vi "IntegStart.vi"(0 "Time step":dbl format="%#_13g", 1 "Generator frequency":dbl, 2 "Number of ignored periods":i32, 3 "Field":dbl[](array[numeric]), 4 "BH averages":i32) -> (5 "Min Index":i32[](array[numeric]), 6 "Max Index":i32[](array[numeric]))   [LabVIEW 2015]
uses:
  <vilib>/express/express arith-compare/Formula/XNode/ExpressFormulaBlockNode.xnode
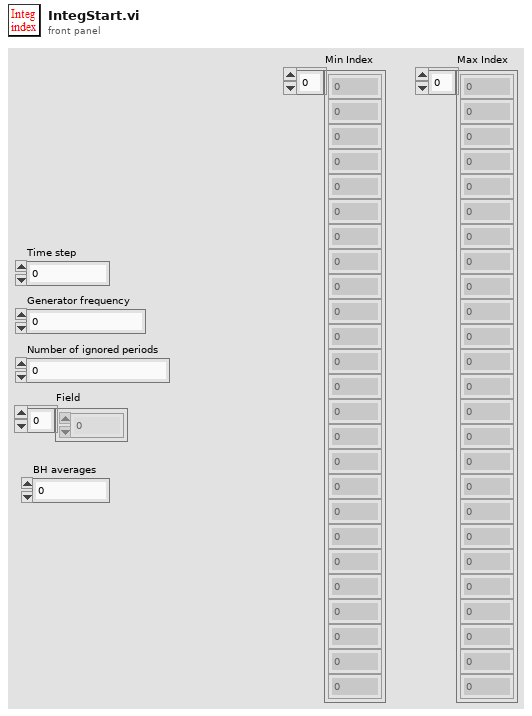
[diagram p1: front panel]
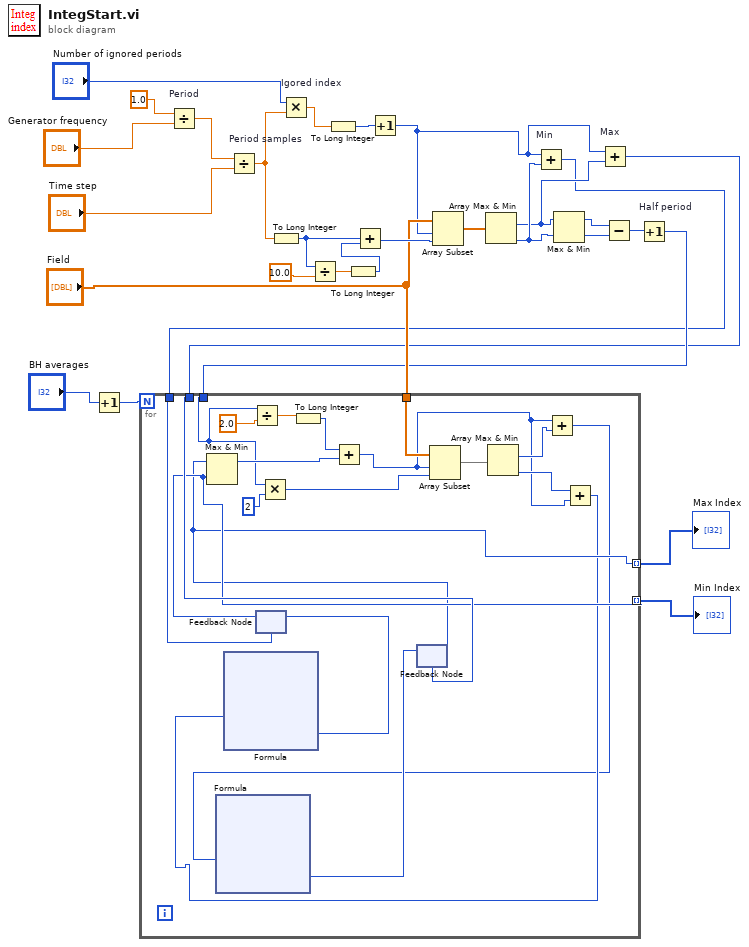
[diagram p0: block diagram]
diagram:
  n1 = Increment(x="BH averages") -> (x+1=w5:i32)
  n2 = Divide "Period"(x=1.0, y="Generator frequency") -> (x/y=w18:dbl)
  n3 = Divide "Period samples"(x=w18, y="Time step") -> (x/y=w19:dbl)
  n4 = To Long Integer(number=w19) -> (32bit integer=w16:i32)
  n5 = Multiply "Igored index"(x="Number of ignored periods", y=w19) -> (x*y=w23:dbl)
  n6 = Divide(x=w16, y=10.0) -> (x/y=w15:dbl)
  n7 = To Long Integer(number=w23) -> (32bit integer=w20:i32)
  n8 = To Long Integer(number=w15) -> (32bit integer=w14:i32)
  n9 = Add(x=w16, y=w14) -> (x+y=w13:i32)
  n10 = Increment(x=w20) -> (x+1=w9:i32)
  n11 = Array Subset(array="Field", index=w9, length=w13) -> (w24:dbl[])
  n12 = Array Max & Min(array=w24) -> (max index (indices)=w8:i32, min index (indices)=w10:i32)  [unwired: 2 out]
  n13 = Add "Min"(x=w9, y=w10) -> (x+y=w2:i32)
  n14 = Max & Min(x=w8, y=w10) -> (max(x,y)=w22:i32, min(x,y)=w21:i32)
  n15 = Add "Max"(x=w9, y=w8) -> (x+y=w1:i32)
  n16 = Subtract(x=w22, y=w21) -> (x-y=w12:i32)
  n17 = Increment "Half period"(x=w12) -> (x+1=w3:i32)
  n18 = for {
    N: w5 -> [_]
    tunnel: "Field" -> [w48]
    tunnel: [w32] -> w6 mode=indexing
    tunnel: [w31] -> w7 mode=indexing
    tunnel: w3 -> [w40]
    tunnel: w1 -> [w33]
    tunnel: w2 -> [w35]
    n19 = Divide(x=w40, y=2.0) -> (x/y=w45:dbl)
    n20 = feedback #1(w35) -> (w32:i32)
    n21 = Multiply(x=w40, y=2) -> (x*y=w42:i32)
    n22 = To Long Integer(number=w45) -> (32bit integer=w44:i32)
    n23 = feedback #2(w33) -> (w31:i32)
    n24 = Max & Min(x=w31, y=w32) -> (max(x,y)=w41:i32)  [unwired: 1 out]
    n25 = Add(x=w44, y=w41) -> (x+y=w37:i32)
    n26 = Array Subset(array=w48, index=w37, length=w42) -> (w47:dbl[])
    n27 = Array Max & Min(array=w47) -> (max index (indices)=w39:i32, min index (indices)=w38:i32)  [unwired: 2 out]
    n28 = Add(x=w37, y=w39) -> (x+y=w29:i32)
    n29 = xnode "Formula"("X1"=w29) -> ("Result"=w34:i32)  [unwired: 1 in, 1 out]
    n30 = feedback-in #2(w34) -> ()
    n31 = Add(x=w38, y=w37) -> (x+y=w30:i32)
    n32 = xnode "Formula"("X1"=w30) -> ("Result"=w36:i32)  [unwired: 1 in, 1 out]
    n33 = feedback-in #1(w36) -> ()
  }
  "Max Index" <- w7
  "Min Index" <- w6
